vi "get_node_updated_object.vi"(0 "node":u8, 5 "index":u16, 7 "subind":u8, 9 "num":u64) -> (4 "return":i16, 6 "node":u8, 8 "index":u16, 10 "subind":u8, 15 "num":u64)   [LabVIEW 2011]
uses:
  canopen_dll_master.dll
panel:
  in  "num":cluster{"num":u64}
  in  "subind":cluster{"subind":u8}
  in  "index":cluster{"index":u16}
  in  "node":cluster{"node":u8}
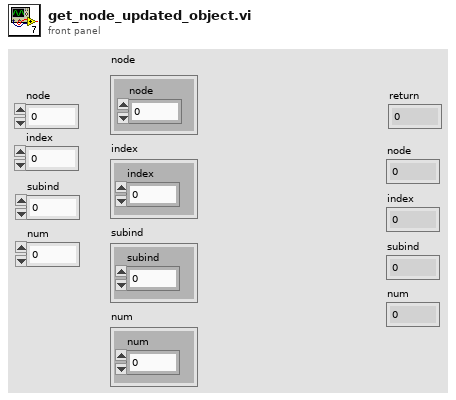
[diagram p1: front panel]
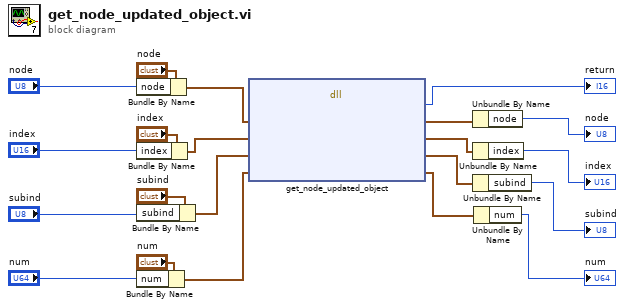
[diagram p0: block diagram]
diagram:
  n1 = Bundle By Name(cluster="node", "node"="node") -> (w17:cluster{"node":u8})
  n2 = Bundle By Name(cluster="index", "index"="index") -> (w16:cluster{"index":u16})
  n3 = Bundle By Name(cluster="subind", "subind"="subind") -> (w15:cluster{"subind":u8})
  n4 = Bundle By Name(cluster="num", "num"="num") -> (w14:cluster{"num":u64})
  n5 = dll-call lib="canopen_dll_master.dll" fn="get_node_updated_object"("node"=w17, "index"=w16, "subind"=w15, "num"=w14) -> ("return type"=→"return":i16, "node"=w8:cluster{"node":u8}, "index"=w6:cluster{"index":u16}, "subind"=w4:cluster{"subind":u8}, "num"=w2:cluster{"num":u64})  [unwired: 3 in, 2 out]
  n6 = Unbundle By Name(w8) -> ("node"=→"node":u8)
  n7 = Unbundle By Name(w6) -> ("index"=→"index":u16)
  n8 = Unbundle By Name(w4) -> ("subind"=→"subind":u8)
  n9 = Unbundle By Name(w2) -> ("num"=→"num":u64)
